vi "DualXDCRFolderPrep.vi"(10 "Array in":T1(array[cluster]), 11 "TempPath":path) -> (2 "DualXdcrDataOut":string[](array[string]), 3 "NormalScanDataOut":string[](array[string]))   [LabVIEW 2022 SP3]
uses:
  Switch Modules/SwitchGlobals.vi
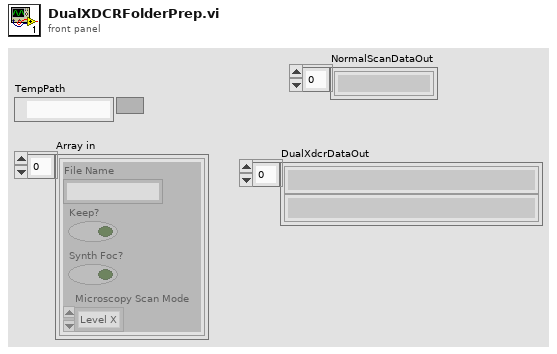
[diagram p1: front panel]
types:
  T1 = cluster{"File Name":string, "Keep?":bool, "Synth Foc?":bool, "Microscopy Scan Mode":enum32{"Level X", "Level Y", "Overview Scan", "Detailed Scan", "V-Z Scan"}}[]
  T2 = typedef "Dual XDCR Complete Settings.ctl" = cluster{"Scan Size":dbl[], "XDCR Offset":dbl[], "Found Home":bool, "XDCR Settings":T3[]}
  T3 = typedef "XDCRSettings.ctl" = cluster{"Transducer Name":string, "Motion Settings":cluster{"Distance between\nscan lines (um)":sgl, "Distance between\nscan planes (um)":sgl}, "Digitizer Settings":cluster{"RF data Sampling":cluster{"Sampling Rate":dbl, "Ref Delay (ms)":dbl, "rf points per line":i32}, "Time scale per Div":dbl, "Voltage Scale":dbl, "Additional dig delay (ms)":dbl}, "Filter Prams":cluster{"low cutoff":i32, "order":i32, "high cutoff":i32}, "XDCR Focal Length":dbl, "Data Vertical Center":dbl, "Image Vertical Offset":dbl, "Daxsonics Settings":T4, "Panametrics Settings":T5, "JSR Complete":T6, "UT340 Controls":T21}
  T4 = typedef "Dax_Control_Cluster.ctl" = cluster{"Freq (MHz) ":u16, "Voltage (V)":u16, "Gain (dB)":u16}
  T5 = typedef "Pana5900.ctl" = cluster{"ENERGY (uJ)":u16, "DAMPING (Ohm)":u16, "HP FILT (KHz) ":u16, "LP FILT (MHz)":u16, "MODE":u16, "PRF (KHz)":u16, "GAIN (db)":u16, "COARSE ATTENUATION":u16, "FINE ATTENUATION":u16}
  T6 = typedef "JSR Complete.ctl" = cluster{"JSR Pulse Settings":T7, "JSR Receive Settings":T12, "JSR Trigger Settings":T17}
  T7 = typedef "JSR Pulse.ctl" = cluster{"Damping":T8, "Pulse Energy Level":T9, "Pulser Impedance":T10, "Pulser Voltage (V)":T11}
  T8 = typedef "Damping.ctl" = i16
  T9 = typedef "Energy.ctl" = u16
  T10 = typedef "Z.ctl" = u16
  T11 = typedef "Volt.ctl" = i16
  T12 = typedef "JSR Recieve.ctl" = cluster{"Receiver Mode":T13, "High Pass Filter":T14, "Low Pass Filter":T15, "Gain (dB)":T16}
  T13 = typedef "Mode.ctl" = i8
  T14 = typedef "HPF.ctl" = u16
  T15 = typedef "LPF.ctl" = u16
  T16 = typedef "Gain.ctl" = i8
  T17 = typedef "JSR Trigger.ctl" = cluster{"External Trigger Limit":T18, "Trigger Source":T19, "PRF (Hz)":T20}
  T18 = typedef "Trig Limit.ctl" = i8
  T19 = typedef "Trig Source.ctl" = i8
  T20 = typedef "PRF.ctl" = dbl
  T21 = typedef "UTEX Controls.ctl" = cluster{"High Pass On":bool, "High Pass Filter (MHz)":i16, "Low Pass On":bool, "Low Pass Filter (MHz)":i16, "PE Gain (dB)":i16, "Voltage":i16, "Pulse Width (ns)":dbl, "Mode":bool, "PC Gain (dB)":i16, "Trig Source":bool, "Rep Rate (Hz)":i16, "PULSE":bool}
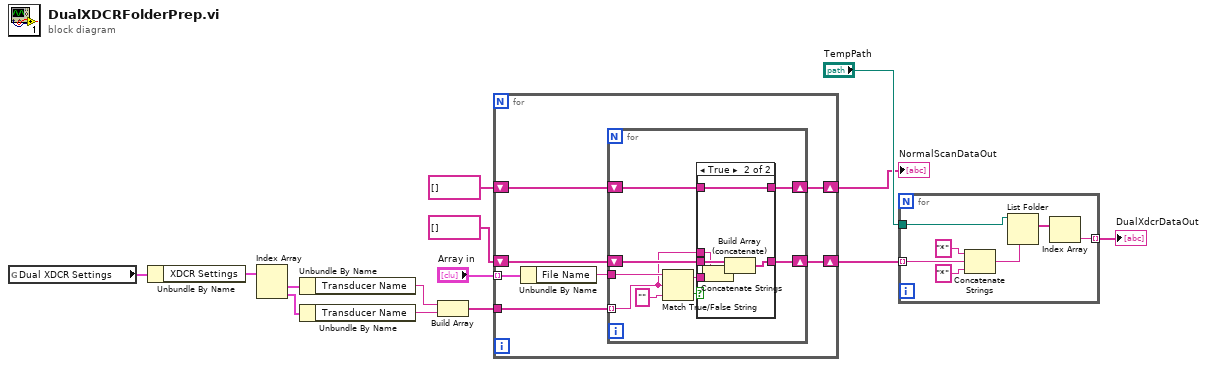
[diagram p0: block diagram]
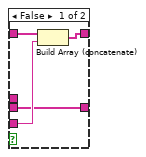
[diagram p2: hidden frame]
diagram:
  n1 = global read "SwitchGlobals.vi" "Dual XDCR Settings"() -> (w5:T2)
  n2 = Unbundle By Name(w5) -> ("XDCR Settings"=w6:T3[])
  n3 = Index Array(array=w6) -> (element #1=w7:T3, element #2=w8:T3)  [unwired: 2 in]
  n4 = Unbundle By Name(w7) -> ("Transducer Name"=w9:string)
  n5 = Unbundle By Name(w8) -> ("Transducer Name"=w10:string)
  n6 = Build Array(w9, w10) -> (w11:string[])
  n7 = for {
    tunnel: "Array in" -> [w19] mode=indexing
    tunnel: w11 -> [w20]
    shift-right: [w17] -> w13
    shift-left: string[] [] ("File Name") -> [w18]
    shift-right: [w15] -> w1
    shift-left: string[] [] ("File Name") -> [w16]
    n8 = Unbundle By Name(w19) -> ("File Name"=w21:string)
    n9 = for {
      tunnel: w21 -> [w30]
      tunnel: w20 -> [w22] mode=indexing
      shift-right: [w25] -> w17
      shift-left: w18 -> [w27]
      shift-right: [w23] -> w15
      shift-left: w16 -> [w24]
      n10 = Match True/False String(2:"" ("false string"), 3:w22, 4:w30) -> (0:w28:bool, 1:w26:string)
      n11 = case shown="True" w28 {
        tunnel: [w31 w39] -> w25
        tunnel: w27 -> [w31 w40]
        tunnel: w26 -> [w34 w38]
        tunnel: w24 -> [w33 w37]
        tunnel: [w32 w37] -> w23
        tunnel: w22 -> [_ w35]
        frame False {
          n12 = Build Array (concatenate)(w33, w34) -> (w32:string[])
        }
        frame True {
          n13 = Concatenate Strings(w35, w38) -> (w36:string)
          n14 = Build Array (concatenate)(w40, w36) -> (w39:string[])
        }
      }
    }
  }
  "NormalScanDataOut" <- w1
  n15 = for {
    tunnel: "TempPath" -> [w47]
    tunnel: w13 -> [w42] mode=indexing
    tunnel: [w41] -> w14 mode=indexing
    n16 = Concatenate Strings("*", w42, "*") -> (w45:string)
    n17 = List Folder(path=w47, pattern=w45) -> (filenames=w46:string[])  [unwired: 1 in, 4 out]
    n18 = Index Array(array=w46) -> (element=w41:string)  [unwired: 1 in]
  }
  "DualXdcrDataOut" <- w14
